vi "Hindbrain.vi"(7 "Notifiers":T1, 8 "XBEE Refference":refnum<visa-resource-name>) -> (3 "String Received":string)   [LabVIEW 2012]
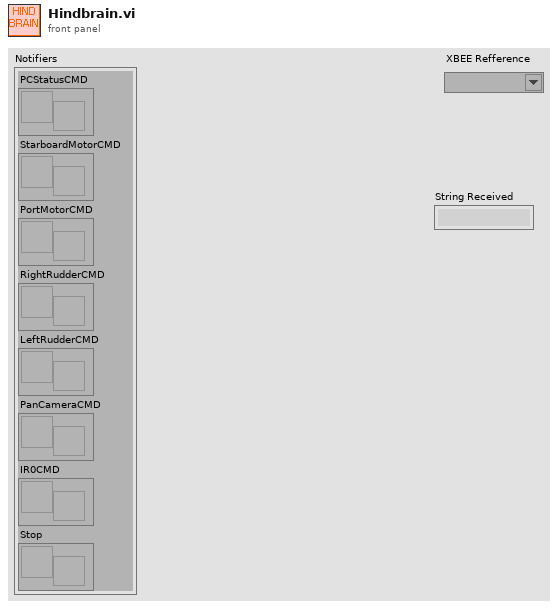
[diagram p1: front panel]
types:
  T1 = cluster{"PCStatusCMD":refnum<notifier>, "StarboardMotorCMD":refnum<notifier>, "PortMotorCMD":refnum<notifier>, "RightRudderCMD":refnum<notifier>, "LeftRudderCMD":refnum<notifier>, "PanCameraCMD":refnum<notifier>, "IR0CMD":refnum<notifier>, "Stop":refnum<notifier>}
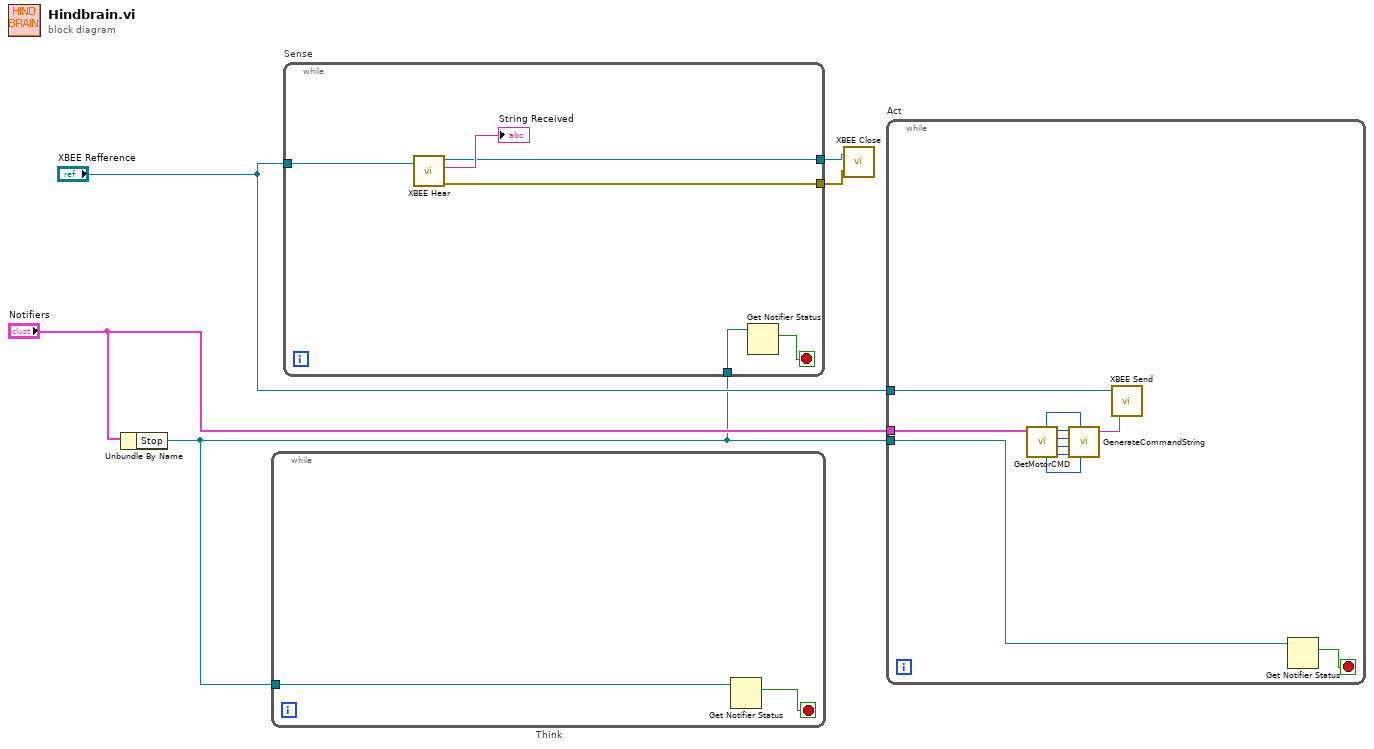
[diagram p0: block diagram]
diagram:
  n1 = Unbundle By Name("Notifiers") -> ("Stop"=w3:refnum<notifier>)
  n2 = while "Think" {
    tunnel: w3 -> [w6]
    stop <- w7 stop-if-true
    n3 = Get Notifier Status(notifier=w6) -> (current notification=w7:bool)  [unwired: 1 in, 4 out]
  }
  n4 = while "Sense" {
    tunnel: "XBEE Refference" -> [w13]
    tunnel: w3 -> [w11]
    tunnel: [w9] -> w2
    tunnel: [w8] -> w1
    stop <- w12 stop-if-true
    n5 = call "XBEE Hear.vi"("VISA resource name"=w13) -> ("VISA resource name out"=w9:refnum<visa-resource-name>, "String Received"=→"String Received":string, "error out"=w8:errorcluster)  [unwired: 1 in, 1 out]
    n6 = Get Notifier Status(notifier=w11) -> (current notification=w12:bool)  [unwired: 1 in, 4 out]
  }
  n7 = call "XBEE Close.vi"("error in (no error)"=w1, "VISA resource name"=w2) -> ()
  n8 = while "Act" {
    tunnel: "XBEE Refference" -> [w24]
    tunnel: "Notifiers" -> [w16]
    tunnel: w3 -> [w14]
    stop <- w15 stop-if-true
    n9 = call "GetMotorCMD.vi"("Notifiers"=w16) -> ("PanCameraCMD"=w23:i32, "LeftRudderCMD"=w22:i32, "StarboardMotorCMD"=w21:i32, "PCStatusCMD"=w20:i32, "RightRudderCMD"=w18:i32, "PortMotorCMD"=w19:i32)  [unwired: 5 in]
    n10 = call "GenerateCommandString.vi"("PC Status"=w20, "Port\nMotor"=w19, "Starboard\nMotor"=w21, "Left Rudder"=w22, "Right Rudder"=w18, "Pan Camera"=w23) -> ("CommandString"=w17:string)  [unwired: 2 in]
    n11 = call "XBEE Send.vi"("String"=w17, "VISA resource name"=w24) -> ()  [unwired: 1 in, 3 out]
    n12 = Get Notifier Status(notifier=w14) -> (current notification=w15:bool)  [unwired: 1 in, 4 out]
  }
